vi "test.network.ipReporter.vi"() -> ()   [LabVIEW 2017]
uses:
  Network/IP Reporter/_Typedef/Def-IniSettings -- Cluster.ctl
  <userlib>/_MGI/Application Control/MGI Change Detector/MGI Change Detector (T).vi
panel:
  in  "notification":string
  in  "stop":bool
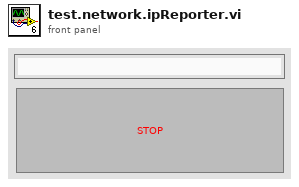
[diagram p1: front panel]
types:
  T1 = typedef "Def-IniSettings -- Cluster.ctl" = cluster{"address":string, "receiver port":u16, "Ignore Gateway IP":bool, "HostName":string}
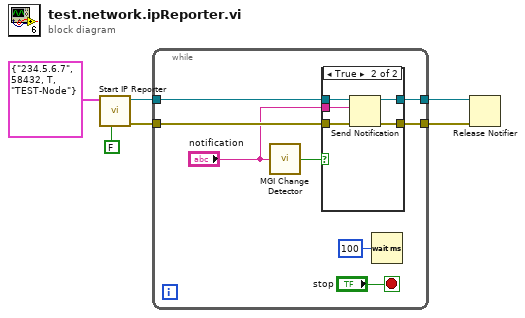
[diagram p0: block diagram]
diagram:
  n1 = call "Start IP Reporter.vi"("Load From File(F)"=FALSE, "Setttings"=T1 {"address"="234.5.6.7", "receiver port"=58432, "Ignore Gateway IP"=TRUE, "HostName"="TEST-Node"}) -> ("error out"=w5:errorcluster, "Information Notifier"=w3:refnum<notifier>)  [unwired: 8 in]
  n2 = while {
    tunnel: w5 -> [w11]
    tunnel: w3 -> [w12]
    tunnel: [w10] -> w2
    tunnel: [w9] -> w1
    stop <- "stop" stop-if-true
    n3 = call-poly <userlib>:"MGI Change Detector.vi"("Value"="notification") -> ("Changed?"=w7:bool)
    n4 = case shown="True" w7 {
      tunnel: w12 -> [w16 w21]
      tunnel: w11 -> [w15 w20]
      tunnel: [w16 w19] -> w10
      tunnel: [w15 w18] -> w9
      tunnel: "notification" -> [_ w17]
      frame False {
      }
      frame True {
        n5 = Send Notification(notification=w17, notifier=w21, error in (no error)=w20) -> (notifier out=w19:refnum<notifier>, error out=w18:errorcluster)
      }
    }
    n6 = Wait (ms)(milliseconds to wait=u32 100) -> ()  [unwired: 1 out]
  }
  n7 = Release Notifier(notifier=w2, error in (no error)=w1) -> ()  [unwired: 1 in, 3 out]
